vi "Main-active object event.vi"() -> ()   [LabVIEW 2019]
uses:
  Active object Event_class/Active object Event.lvclass
panel:
  in  "stop":bool
  in  "ShowProcessWindow":bool
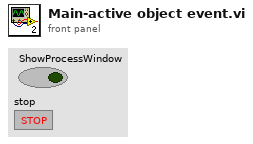
[diagram p1: front panel]
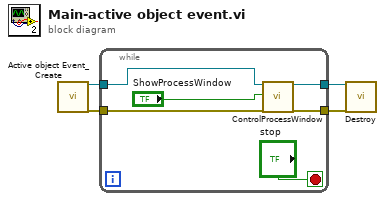
[diagram p0: block diagram]
diagram:
  n1 = call "Active object Event_Create.vi"() -> ("reference out"=w1:refnum<class "Active object Event.lvclass">, "error out"=w4:errorcluster)  [unwired: 18 in]
  n2 = while {
    tunnel: w4 -> [w7]
    tunnel: [w10] -> w3
    tunnel: [w9] -> w2
    tunnel: w1 -> [w8]
    stop <- "stop" stop-if-true
    n3 = call "ControlProcessWindow.vi"("reference in"=w8, "ShowProcessWindow"="ShowProcessWindow", "error in (no error)"=w7) -> ("reference out"=w9:refnum<class "Active object Event.lvclass">, "error out"=w10:errorcluster)  [unwired: 15 in]
  }
  n4 = call-dynamic "Destroy.vi"("reference in"=w2, "error in (no error)"=w3) -> ()  [unwired: 16 in, 2 out]
